vi "test_interp_stage1.vi"() -> ()   [LabVIEW 2013]
uses:
  <vilib>/measure/maspectr.llb/Power Spectrum and PSD Export Mode.ctl
  <vilib>/measure/maspectr.llb/FFT Power Spectrum and PSD for 1 Chan.vi
  <vilib>/measure/NI_MABase.lvlib
  <vilib>/measure/NI_MAPro.lvlib
panel:
  out "Waveform Graph out":dbl[](graph)
  out "Power spectrum in":cluster{"f0":dbl, "df":dbl, "magnitude":dbl[]}(graph)
  out "Power spectrum":cluster{"f0":dbl, "df":dbl, "magnitude":dbl[]}(graph)
  out "Waveform Graph":dbl[](graph)
  out "# of Iterations":i32
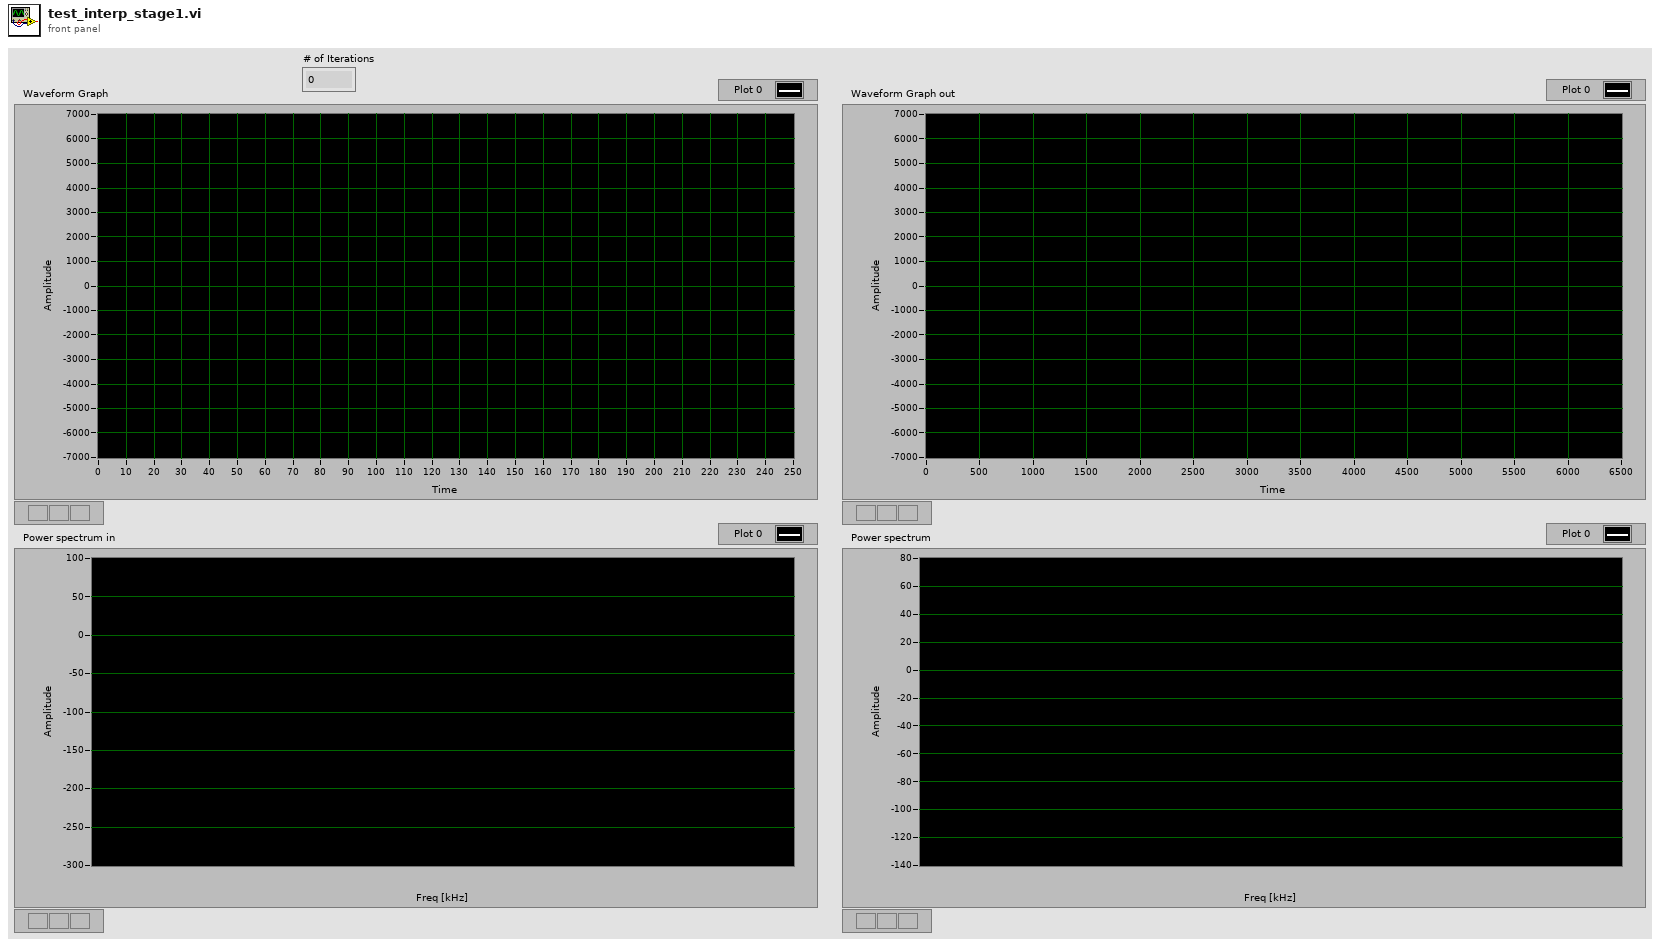
[diagram p1: front panel]
types:
  T1 = typedef "NI_MAPro.lvlib/Power Spectrum and PSD Export Mode.ctl" = u16
  T2 = cluster{"frequency":dbl, "amplitude":dbl, "phase":dbl}[]
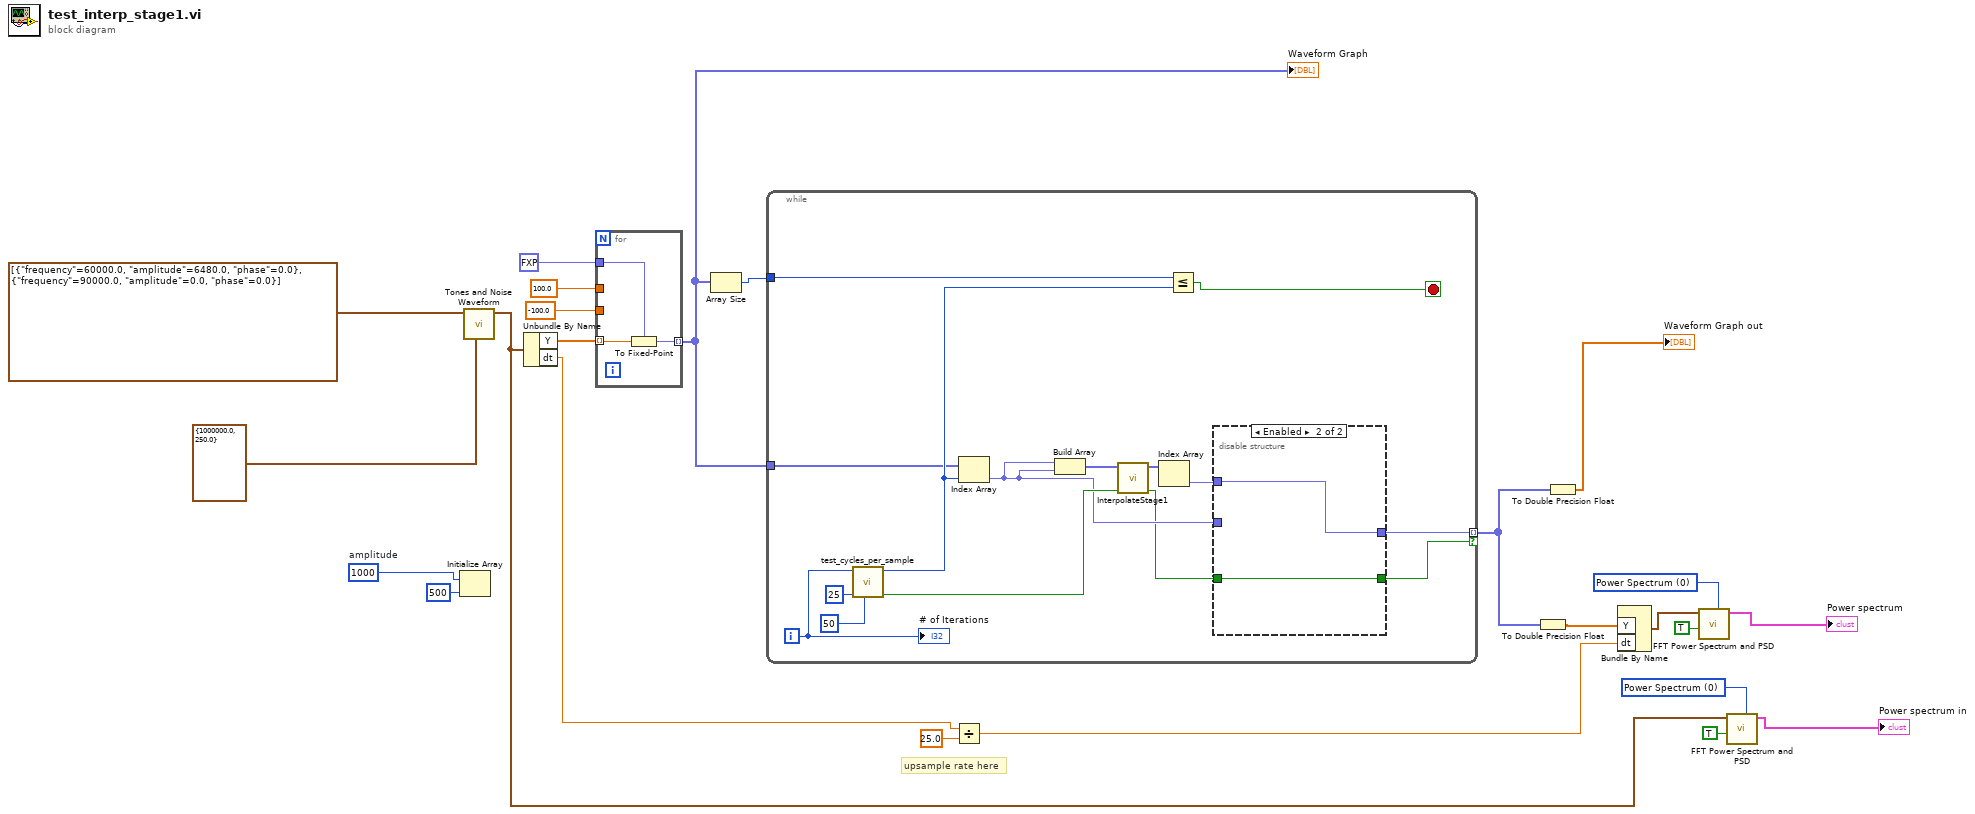
[diagram p0: block diagram]
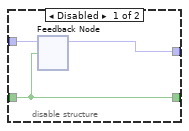
[diagram p2: hidden frame]
diagram:
  w2 = 1000  # amplitude
  w12 = T1 0 items=["Power Spectrum", "Power Spectral Density"] ("export mode")
  w20 = T1 0 items=["Power Spectrum", "Power Spectral Density"] ("export mode")
  # "upsample rate here"
  n1 = Initialize Array(w2, 500 ("dimension size")) -> ()  [unwired: 1 out]
  n2 = call <vilib>:"Tones and Noise Waveform.vi"("sampling info"=cluster{"Fs":dbl, "#s":dbl} {"Fs"=1000000.0, "#s"=250.0}, "tones"=T2 [{"frequency"=60000.0, "amplitude"=6480.0, "phase"=0.0}, {"frequency"=90000.0, "amplitude"=0.0, "phase"=0.0}]) -> ("signal out"=w11:waveform(dbl))  [unwired: 8 in, 1 out]
  n3 = Unbundle By Name(w11) -> ("Y"=w1:dbl[], "dt"=w18:dbl)
  n4 = for {
    tunnel: w1 -> [w25] mode=indexing
    tunnel: fxp<+/-,16,14> 0.0 ("fixed-point type") -> [w27]
    tunnel: [w26] -> w4 mode=indexing
    tunnel: 100.0 -> [_]
    tunnel: -100.0 -> [_]
    n5 = To Fixed-Point(fixed-point type=w27, number=w25) -> (fixed-point=w26:fxp<+/-,16,14>)
  }
  "Waveform Graph" <- w4
  n6 = Array Size(array=w4) -> (size(s)=w5:i32)
  n7 = while {
    tunnel: w4 -> [w34]
    tunnel: [w35] -> w9 mode=indexing if=w36
    tunnel: w5 -> [w39]
    i -> [w42]
    stop <- w37 stop-if-true
    n8 = call "test_cycles_per_sample.vi"("initial delay"=50, "cycles per sample"=25, "index"=w42) -> ("valid out"=w33:bool, "array index"=w38:i32)  [unwired: 7 in]
    n9 = Index Array(array=w34, index=w38) -> (element=w32:fxp<+/-,16,14>)
    n10 = Build Array(w32, w32) -> (w31:fxp<+/-,16,14>[])
    n11 = call "InterpolateStage1.vi"("valid in"=w33, "Data in"=w31) -> ("valid out"=w28:bool, "Data out"=w29:fxp<+/-,16,14>[])  [unwired: 8 in]
    n12 = Index Array(array=w29) -> (element=w30:fxp<+/-,16,14>)  [unwired: 1 in]
    n13 = Less Or Equal?(x=w39, y=w38) -> (x <= y?=w37:bool)
    n14 = disable-structure shown="Enabled" {
      disable-tunnel: w32 -> [w45 _]
      disable-tunnel: w28 -> [w44 w46]
      disable-tunnel: [w44 w46] -> w36
      disable-tunnel: [w43 w47] -> w35
      disable-tunnel: w30 -> [_ w47]
      frame Disabled {
        n15 = feedback-in #1(w45, w44) -> ()
        n16 = feedback #1() -> (w43:fxp<+/-,16,14>)  [unwired: 1 in]
      }
      frame Enabled {
      }
    }
    "# of Iterations" <- w42
  }
  n17 = Divide(x=w18, y=25.0) -> (x/y=w16:dbl)
  n18 = To Double Precision Float(number=w9) -> (double precision float=w14:dbl[])
  n19 = To Double Precision Float(number=w9) -> (double precision float=→"Waveform Graph out":dbl[])
  n20 = Bundle By Name("Y"=w14, "dt"=w16) -> (w21:waveform(dbl))  [unwired: 1 in]
  n21 = call-poly <vilib>:"FFT Power Spectrum and PSD.vi"("export mode"=w20, "dB On (F)"=TRUE, "time signal"=w21) -> ("Power Spectrum / PSD"=→"Power spectrum":cluster{"f0":dbl, "df":dbl, "magnitude":dbl[]})  [unwired: 5 in, 3 out]
  n22 = call-poly <vilib>:"FFT Power Spectrum and PSD.vi"("export mode"=w12, "dB On (F)"=TRUE, "time signal"=w11) -> ("Power Spectrum / PSD"=→"Power spectrum in":cluster{"f0":dbl, "df":dbl, "magnitude":dbl[]})  [unwired: 5 in, 3 out]
